vi "FlatToRichnixnet_grpc_EptRxFilter.vi"(5 "OutputClusterType":T1, 11 "InputCluster":T2) -> (3 "OutputCluster":T1)   [LabVIEW 2025, in "xnet-grpc_client.lvlib"]
uses:
  xnet-grpc_client.lvlib
  nixnet_grpc_EptRxFilter_Flat.ctl
  nixnet_grpc_EptRxFilter.ctl
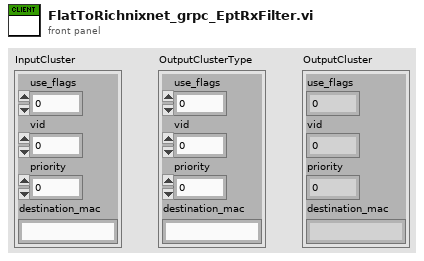
[diagram p1: front panel]
types:
  T1 = typedef "xnet-grpc_client.lvlib/nixnet_grpc_EptRxFilter.ctl" = cluster{"use_flags":u32, "vid":u32, "priority":u32, "destination_mac":string}
  T2 = typedef "xnet-grpc_client.lvlib/nixnet_grpc_EptRxFilter_Flat.ctl" = cluster{"use_flags":u32, "vid":u32, "priority":u32, "destination_mac":string}
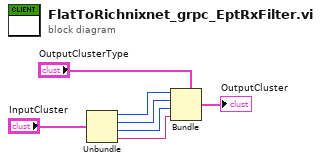
[diagram p0: block diagram]
diagram:
  n1 = Unbundle "Unbundle"("InputCluster") -> ("use_flags"=w4:u32, "vid"=w3:u32, "priority"=w2:u32, "destination_mac"=w1:string)
  n2 = Bundle "Bundle"(cluster="OutputClusterType", "use_flags"=w4, "vid"=w3, "priority"=w2, "destination_mac"=w1) -> (→"OutputCluster":T1)
